vi "Update State Data.vi"(8 "error in (no error)":errorcluster, 9 "Data":variant, 10 "Argument":string, 11 "Numeric Assertion in":refnum<class "Numeric Assertion.lvclass">) -> (0 "error out":errorcluster, 3 "Numeric Assertion out":refnum<class "Numeric Assertion.lvclass">)   [LabVIEW 2020, in "MacroAssert.lvlib" / "Numeric Assertion.lvclass"]
uses:
  Numeric Assertion.lvclass
  Numeric Assertion Type.ctl
  Numeric Comparator.ctl
  Assertion Step/Assertion Step.lvclass
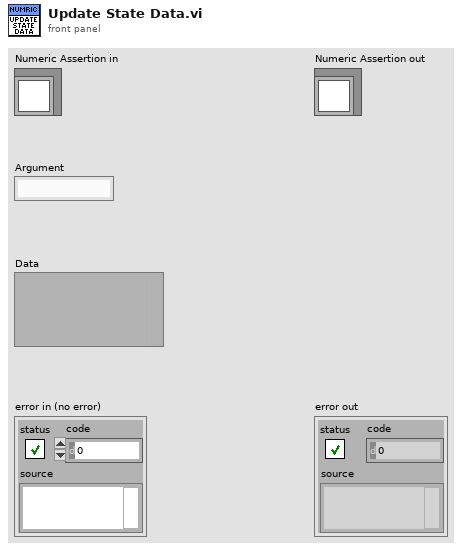
[diagram p1: front panel]
types:
  T1 = typedef "MacroAssert.lvlib/Numeric Assertion.lvclass/Numeric Assertion Type.ctl" = enum16{"Numeric Ctl Value", "Ctl Width Property", "Ctl Height Property", "VI Width", "VI Height", "Window Width", "Window Height"}
  T2 = typedef "MacroAssert.lvlib/Numeric Assertion.lvclass/Numeric Comparator.ctl" = enum16{"Equals", "Is greater than", "Is greater than or equal to", "Is less than", "Is less than or equal to", "Does not equal"}
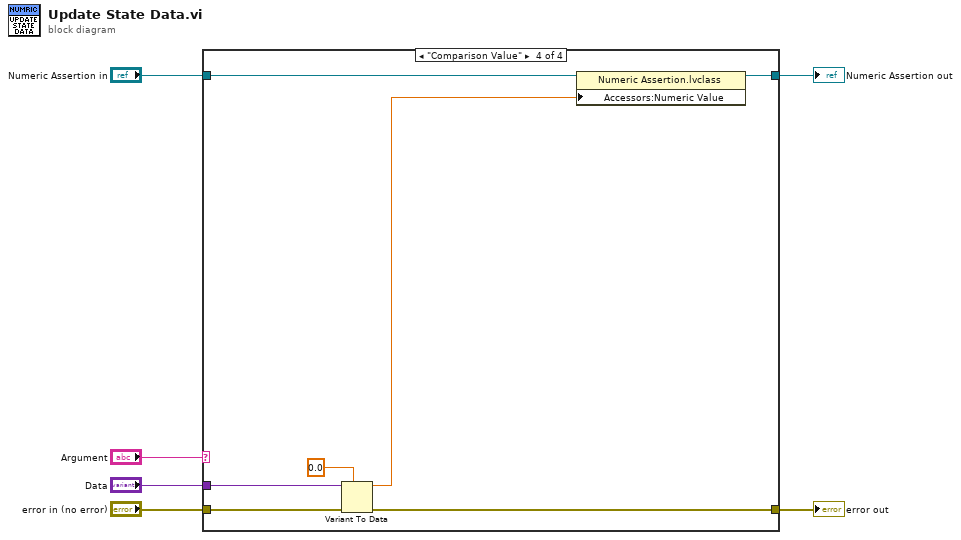
[diagram p0: block diagram]
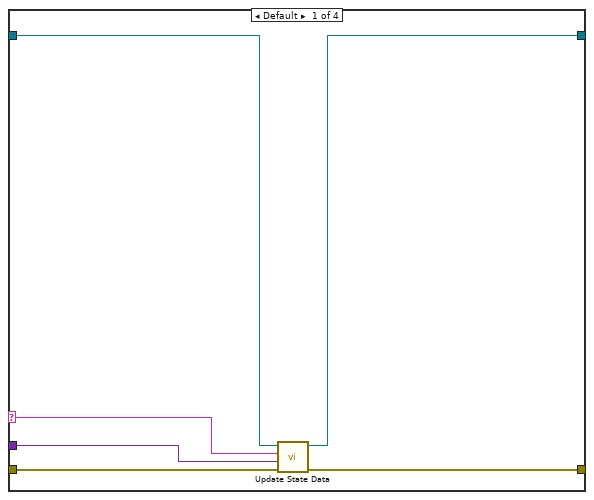
[diagram p2: hidden frame]
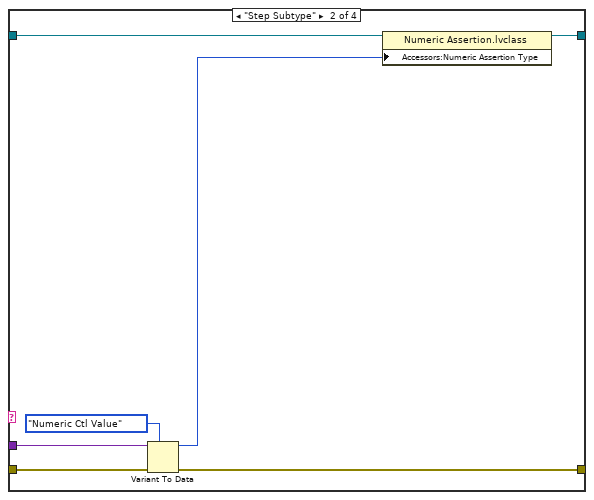
[diagram p3: hidden frame]
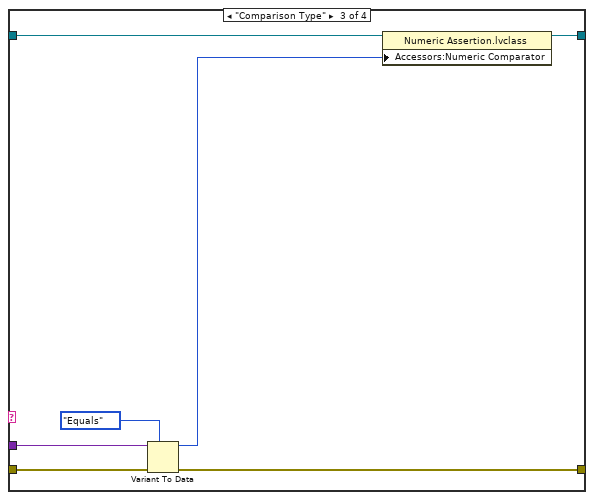
[diagram p4: hidden frame]
diagram:
  n1 = case shown="\"Comparison Value\"" "Argument" {
    selector: "Argument" -> [w9 _ _ _]
    tunnel: "Numeric Assertion in" -> [w8 w19 w26 w33]
    tunnel: "error in (no error)" -> [w12 w17 w24 w31]
    tunnel: [w7 w18 w25 w32] -> w2
    tunnel: [w11 w16 w23 w30] -> w1
    tunnel: "Data" -> [w10 w14 w22 w29]
    frame Default {
      n2 = call-parent "Update State Data.vi"("error in (no error)"=w12, "Data"=w10, "Argument"=w9, "Assertion Step in"=w8) -> ("error out"=w11:errorcluster, "Assertion Step out"=w7:refnum<class "Numeric Assertion.lvclass">)  [unwired: 6 in]
    }
    frame "Step Subtype" {
      n3 = Variant To Data(error in=w17, type=Numeric_Assertion_Type."Numeric Ctl Value" ("Numeric Assertion Type"), Variant=w14) -> (data=w13:T1, error out=w16:errorcluster)
      n4 = property class="Numeric Assertion.lvclass"(reference=w19, "Accessors:Numeric Assertion Type"=w13) -> (reference out=w18:refnum<class "Numeric Assertion.lvclass">)  [unwired: 1 in, 1 out]
    }
    frame "Comparison Type" {
      n5 = Variant To Data(error in=w24, type=Numeric_Comparator."Equals" ("Numeric Comparator"), Variant=w22) -> (data=w21:T2, error out=w23:errorcluster)
      n6 = property class="Numeric Assertion.lvclass"(reference=w26, "Accessors:Numeric Comparator"=w21) -> (reference out=w25:refnum<class "Numeric Assertion.lvclass">)  [unwired: 1 in, 1 out]
    }
    frame "Comparison Value" {
      n7 = Variant To Data(error in=w31, type=0.0, Variant=w29) -> (data=w28:dbl, error out=w30:errorcluster)
      n8 = property class="Numeric Assertion.lvclass"(reference=w33, "Accessors:Numeric Value"=w28) -> (reference out=w32:refnum<class "Numeric Assertion.lvclass">)  [unwired: 1 in, 1 out]
    }
  }
  "error out" <- w1
  "Numeric Assertion out" <- w2
